vi "Init_PCI6602_Counter.vi"(4 "error in":errorcluster, 5 "Main cluster":T1, 6 "Acquisition time (s)":dbl, 7 "Device":tag="APD_Count") -> (0 "error out":errorcluster, 1 "Main cluster":T1, 2 "Clock task":refnum<k21>, 3 "Counter task":refnum<k21>)   [LabVIEW 2010]
uses:
  Main_cluster.ctl
  <vilib>/vision/Image Controls.llb/IMAQ Image.ctl
  <vilib>/DAQmx/create/channels.llb/DAQmx Create Channel (CI-Count Edges).vi
  <vilib>/DAQmx/create/channels.llb/DAQmx Create Channel (CO-Pulse Generation-Frequency).vi
  <vilib>/DAQmx/configure/timing.llb/DAQmx Timing (Implicit).vi
  <vilib>/DAQmx/configure/timing.llb/DAQmx Timing (Sample Clock).vi
  <vilib>/DAQmx/create/channels.llb/DAQmx Create Channel (AO-Voltage-Basic).vi
  C:/Program Files (x86)/National Instruments/LabVIEW 2010/resource/objmgr/daqmx.rc
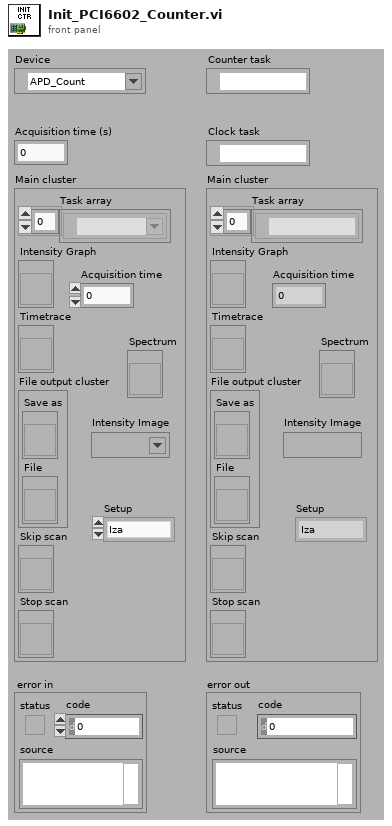
[diagram p1: front panel]
types:
  T1 = typedef "Main_cluster.ctl" = cluster{"Task array":refnum<k21>[], "Intensity Graph":refnum<vi>, "Timetrace":refnum<vi>, "File output cluster":cluster{"Save as":refnum<vi>, "File":refnum<vi>}, "Skip scan":refnum<vi>, "Stop scan":refnum<vi>, "Acquisition time":dbl, "Setup":enum16{"Iza", "Lukasz"}, "Spectrum":refnum<vi>, "Intensity Image":T2}
  T2 = typedef "IMAQ Image.ctl" = refnum<image>
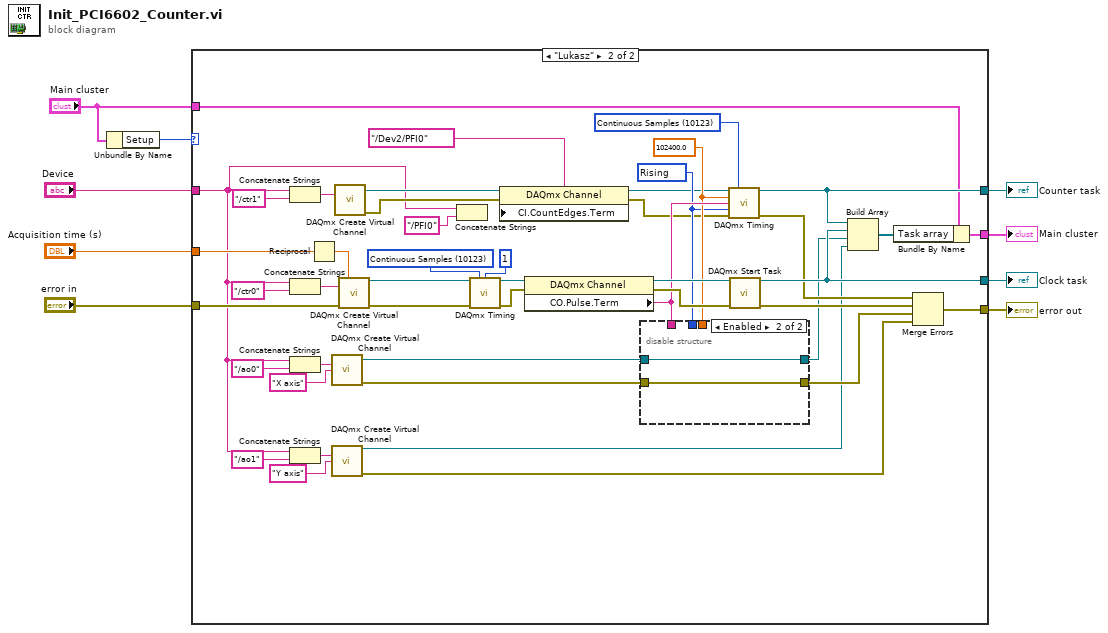
[diagram p0: block diagram]
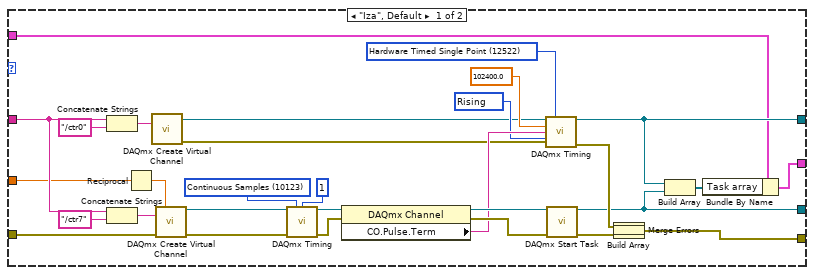
[diagram p2: hidden frame]
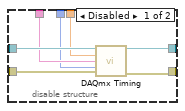
[diagram p3: hidden frame]
diagram:
  n1 = Unbundle By Name("Main cluster") -> ("Setup"=w1:enum16{"Iza", "Lukasz"})
  n2 = case shown="\"Lukasz\"" w1 {
    tunnel: [w36 w83] -> w9
    tunnel: "Device" -> [w24 w42]
    tunnel: "Acquisition time (s)" -> [w19 w71]
    tunnel: "error in" -> [w16 w69]
    tunnel: [w15 w68] -> w5
    tunnel: [w14 w67] -> w4
    tunnel: "Main cluster" -> [w13 w66]
    tunnel: [w11 w64] -> w3
    frame "Iza", Default {
      w33 = 10123 items=["Finite Samples"=10178, "Continuous Samples"=10123, "Hardware Timed Single Point"=12522] ("sample mode")
      w27 = 12522 items=["Finite Samples"=10178, "Continuous Samples"=10123, "Hardware Timed Single Point"=12522] ("sample mode")
      w26 = 10280 items=["Rising"=10280, "Falling"=10171] ("active edge")
      n3 = Concatenate Strings(w24, "/ctr0" ("string")) -> (w21:string)
      n4 = Concatenate Strings(w24, "/ctr7" ("string")) -> (w31:string)
      n5 = Reciprocal(x=w19) -> (1/x=w22:dbl)
      n6 = call-poly <vilib>:"DAQmx Create Virtual Channel.vi"("counter"=w21) -> ("task out"=w17:refnum<k21>, "error out"=w18:errorcluster)  [unwired: 13 in]
      n7 = call-poly <vilib>:"DAQmx Create Virtual Channel.vi"("frequency"=w22, "counter"=w31, "error in"=w16) -> ("task out"=w30:refnum<k21>, "error out"=w34:errorcluster)  [unwired: 11 in]
      n8 = call-poly <vilib>:"DAQmx Timing.vi"("task/channels in"=w30, "sample mode"=w33, "samples per channel"=1, "error in"=w34) -> ("task out"=w32:refnum<k21>, "error out"=w35:errorcluster)  [unwired: 10 in]
      n9 = property class="DAQmx Channel"(reference=w32, error in=w35) -> (reference out=w37:refnum<k21>, error out=w40:errorcluster, "CO.Pulse.Term"=w29:tag)
      n10 = call-poly <vilib>:"DAQmx Timing.vi"("task/channels in"=w17, "sample mode"=w27, "rate"=102400.0, "source"=w29, "active edge"=w26, "error in"=w18) -> ("task out"=w15:refnum<k21>, "error out"=w28:errorcluster)  [unwired: 8 in]
      n11 = call <vilib>:"DAQmx Start Task.vi"("task/channels in"=w37, "error in"=w40) -> ("task out"=w14:refnum<k21>, "error out"=w39:errorcluster)  [unwired: 12 in]
      n12 = Build Array(w28, w39) -> (w10:errorcluster[])
      n13 = Merge Errors(w10) -> (w36:errorcluster)
      n14 = Build Array(w15, w14) -> (w12:refnum<k21>[])
      n15 = Bundle By Name(cluster=w13, "Task array"=w12) -> (w11:T1)
    }
    frame "Lukasz" {
      w80 = 10123 items=["Finite Samples"=10178, "Continuous Samples"=10123, "Hardware Timed Single Point"=12522] ("sample mode")
      w76 = 10123 items=["Finite Samples"=10178, "Continuous Samples"=10123, "Hardware Timed Single Point"=12522] ("sample mode")
      w52 = 10280 items=["Rising"=10280, "Falling"=10171] ("active edge")
      w53 = 102400.0 ("rate")
      n16 = Concatenate Strings(w42, "/ctr1" ("string")) -> (w73:string)
      n17 = Concatenate Strings(w42, "/ctr0" ("string")) -> (w78:string)
      n18 = Concatenate Strings(w42, "/ao0" ("string")) -> (w62:string)
      n19 = Concatenate Strings(w42, "/ao1" ("string")) -> (w50:string)
      n20 = Reciprocal(x=w71) -> (1/x=w74:dbl)
      n21 = call-poly <vilib>:"DAQmx Create Virtual Channel.vi"("physical channels"=w62, "name to assign"="X axis") -> ("task out"=w58:refnum<k21>, "error out"=w59:errorcluster)  [unwired: 12 in]
      n22 = call-poly <vilib>:"DAQmx Create Virtual Channel.vi"("physical channels"=w50, "name to assign"="Y axis") -> ("task out"=w48:refnum<k21>, "error out"=w47:errorcluster)  [unwired: 12 in]
      n23 = call-poly <vilib>:"DAQmx Create Virtual Channel.vi"("counter"=w73) -> ("task out"=w70:refnum<k21>, "error out"=w45:errorcluster)  [unwired: 13 in]
      n24 = call-poly <vilib>:"DAQmx Create Virtual Channel.vi"("frequency"=w74, "counter"=w78, "error in"=w69) -> ("task out"=w77:refnum<k21>, "error out"=w81:errorcluster)  [unwired: 11 in]
      n25 = Concatenate Strings(w42, "/PFI0" ("string")) -> ()  [unwired: 1 out]
      n26 = call-poly <vilib>:"DAQmx Timing.vi"("task/channels in"=w77, "sample mode"=w80, "samples per channel"=1, "error in"=w81) -> ("task out"=w79:refnum<k21>, "error out"=w82:errorcluster)  [unwired: 10 in]
      n27 = property class="DAQmx Channel"(reference=w70, error in=w45, "CI.CountEdges.Term"=tag "/Dev2/PFI0") -> (reference out=w46:refnum<k21>, error out=w44:errorcluster)
      n28 = property class="DAQmx Channel"(reference=w79, error in=w82) -> (reference out=w84:refnum<k21>, error out=w86:errorcluster, "CO.Pulse.Term"=w57:tag)
      n29 = disable-structure shown="Enabled" {
        disable-tunnel: w59 -> [w93 w94]
        disable-tunnel: w58 -> [w92 w95]
        disable-tunnel: w57 -> [w91 _]
        disable-tunnel: [w90 w94] -> w55
        disable-tunnel: [w89 w95] -> w54
        disable-tunnel: w53 -> [w88 _]
        disable-tunnel: w52 -> [w87 _]
        frame Disabled {
          n30 = call-poly <vilib>:"DAQmx Timing.vi"("task/channels in"=w92, "rate"=w88, "source"=w91, "active edge"=w87, "error in"=w93) -> ("task out"=w89:refnum<k21>, "error out"=w90:errorcluster)  [unwired: 9 in]
        }
        frame Enabled {
        }
      }
      n31 = call-poly <vilib>:"DAQmx Timing.vi"("task/channels in"=w46, "sample mode"=w76, "rate"=w53, "source"=w57, "active edge"=w52, "error in"=w44) -> ("task out"=w68:refnum<k21>, "error out"=w61:errorcluster)  [unwired: 8 in]
      n32 = call <vilib>:"DAQmx Start Task.vi"("task/channels in"=w84, "error in"=w86) -> ("task out"=w67:refnum<k21>, "error out"=w60:errorcluster)  [unwired: 12 in]
      n33 = Build Array(w68, w67, w54, w48) -> (w65:refnum<k21>[])
      n34 = Bundle By Name(cluster=w66, "Task array"=w65) -> (w64:T1)
      n35 = Merge Errors(w61, w60, w55, w47) -> (w83:errorcluster)
    }
  }
  "Clock task" <- w4
  "Counter task" <- w5
  "error out" <- w9
  "Main cluster" <- w3
